vi "Set Shutters.vi"(1 "dummy2":i32, 4 "dummy1":i32, 5 "extmode":i32, 6 "exttype":i32, 7 "openingtime":i32, 9 "closingtime":i32, 10 "mode":i32, 11 "typ":i32) -> (3 "function return":u32)   [LabVIEW 2018, in "Copy of Andor SDK.lvlib"]
doc: "EXPNETTYPE unsigned int WINAPI SetShutters(int typ, int mode, int closingtime, int openingtime, int exttype, int extmode, int dummy1, int dummy2);"
uses:
  Copy of Andor SDK.lvlib
  <userlib>/Andor SDK/ATMCD32D.dll
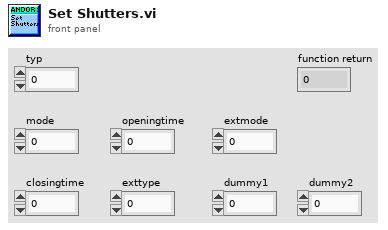
[diagram p1: front panel]
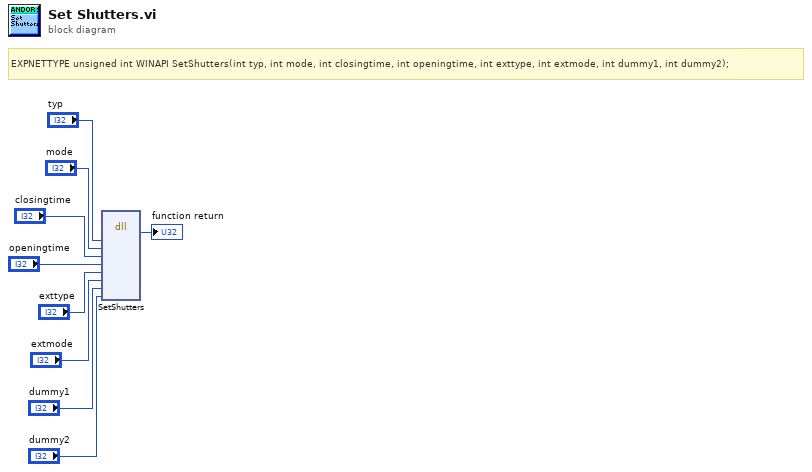
[diagram p0: block diagram]
diagram:
  # "EXPNETTYPE unsigned int WINAPI SetShutters(int typ, int mode, int closingtime, int openingtime, int exttype, int extmode, int dummy1, int dummy2);"
  n1 = dll-call lib="C:/Program Files (x86)/National Instruments/LabVIEW 2018/user.lib/Andor SDK/ATMCD32D.*" fn="SetShutters"("typ"="typ", "mode"="mode", "closingtime"="closingtime", "openingtime"="openingtime", "exttype"="exttype", "extmode"="extmode", "dummy1"="dummy1", "dummy2"="dummy2") -> (→"function return":u32)  [unwired: 11 in, 2 out]
